vi "Remote_call_prep.vi"(3 "Vi Name in":string, 4 "Job Directory In":path, 5 "VI Directory":path) -> (0 "Vi Name out":string, 1 "Job Directory out":path, 2 "cancelled":bool)   [LabVIEW 2021]
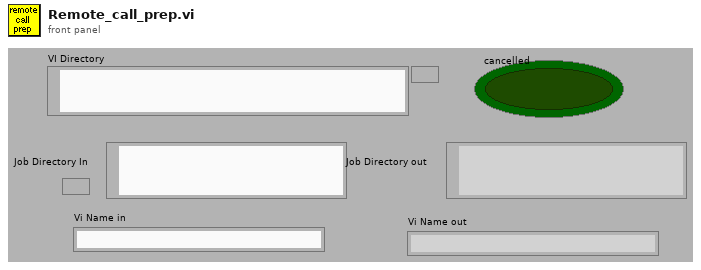
[diagram p1: front panel]
types:
  T1 = enum16{"Zero or one", "One", "Zero or more", "One or more"}
  T2 = enum32{"existing file", "new file", "new or existing file", "existing dir", "new dir", "new or existing dir", "existing file (use LLBs)", "new file (use LLBs)", "new or existing file (use LLBs)", "new or existing file or directory (use LLBs)"}
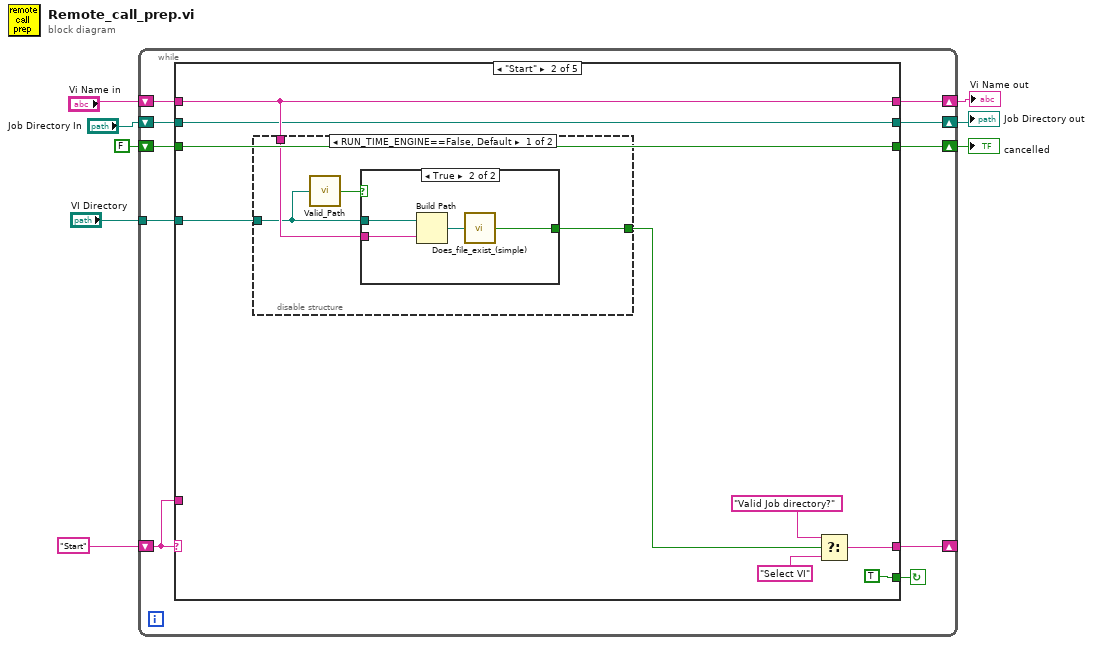
[diagram p0: block diagram]
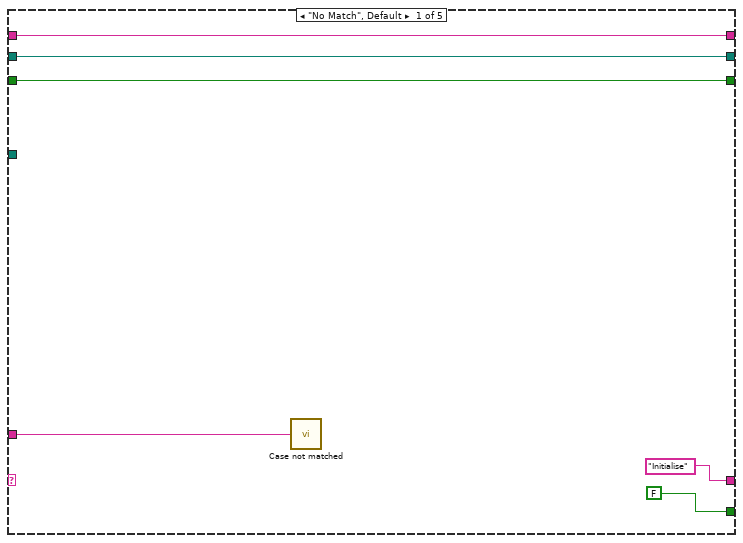
[diagram p2: hidden frame]
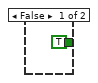
[diagram p3: hidden frame]
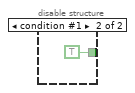
[diagram p4: hidden frame]
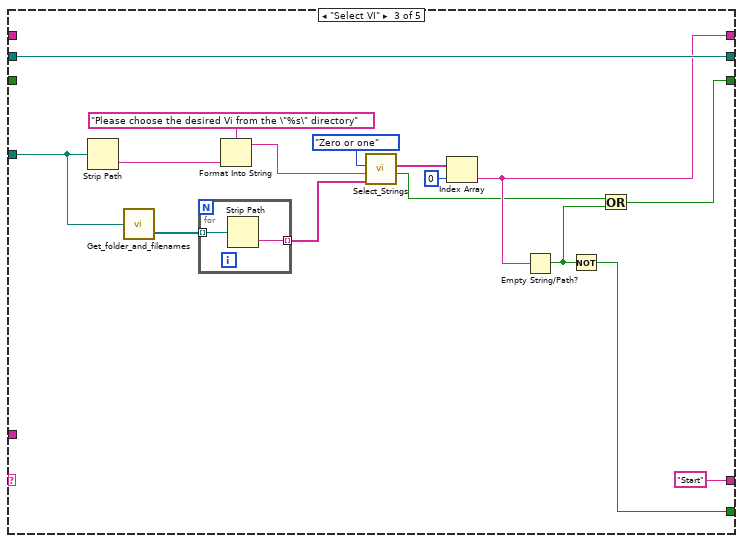
[diagram p5: hidden frame]
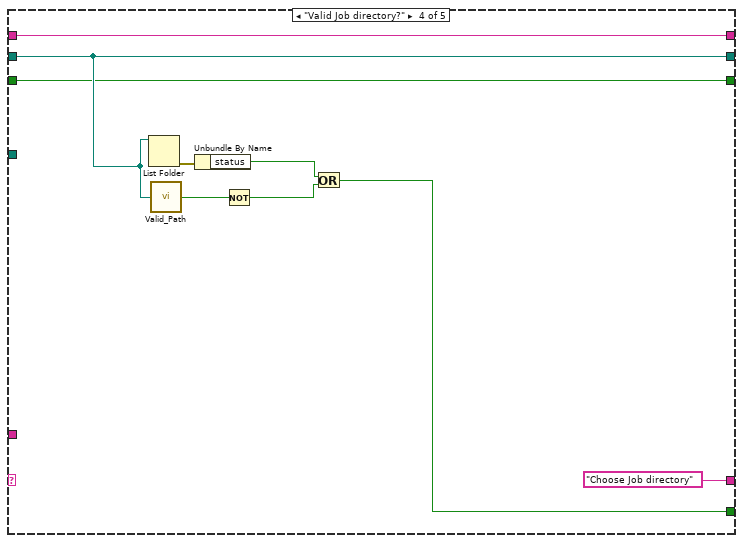
[diagram p6: hidden frame]
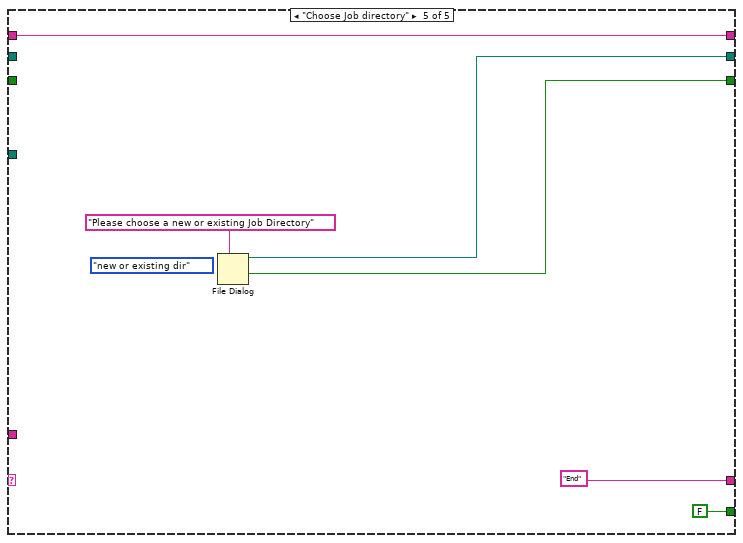
[diagram p7: hidden frame]
diagram:
  n1 = while {
    shift-left: "Start" -> [w16]
    shift-right: [w17] -> _
    tunnel: "VI Directory" -> [w15]
    shift-right: [w13] -> w5
    shift-left: "Vi Name in" -> [w14]
    shift-right: [w11] -> w2
    shift-left: "Job Directory In" -> [w12]
    shift-right: [w10] -> w3
    shift-left: FALSE ("cancelled") -> [w9]
    stop <- w18 continue-if-true
    n2 = case shown="\"Start\"" w16 {
      tunnel: [FALSE TRUE w47 w67 FALSE] -> w18
      tunnel: ["Initialise" w29 "Start" "Choose Job directory" "End"] -> w17
      tunnel: w16 -> [w20 _ _ _ _]
      tunnel: w15 -> [_ w26 w52 _ _]
      tunnel: w14 -> [w22 w28 _ w70 w76]
      tunnel: [w22 w28 w48 w70 w76] -> w13
      tunnel: w12 -> [w21 w27 w53 w68 _]
      tunnel: [w21 w27 w53 w68 w74] -> w11
      tunnel: [w19 w25 w44 w62 w73] -> w10
      tunnel: w9 -> [w19 w25 _ w62 _]
      frame "No Match", Default {
        n3 = call "Case not matched.vi"("Case Name not Matched"=w20) -> ()
      }
      frame "Start" {
        n4 = disable-structure shown="RUN_TIME_ENGINE==False, Default" {
          disable-tunnel: [w37 TRUE ("exists?")] -> w32
          disable-tunnel: w28 -> [w36 _]
          disable-tunnel: w26 -> [w35 _]
          frame condition #0 (active) {
            n5 = call "Valid_Path.vi"("Filename"=w35) -> ("Valid Path?"=w34:bool)
            n6 = case shown="True" w34 {
              tunnel: [TRUE ("exists?") w41] -> w37
              tunnel: w36 -> [_ w40]
              tunnel: w35 -> [_ w39]
              frame False {
              }
              frame True {
                n7 = Build Path(base path=w39, name or relative path=w40) -> (appended path=w42:path)
                n8 = call "Does_file_exist_(simple).vi"("Pathname"=w42) -> ("exists?"=w41:bool)
              }
            }
          }
          frame condition #1 {
          }
        }
        n9 = Select(t="Valid Job directory?", s=w32, f="Select VI") -> (s? t:f=w29:string)
      }
      frame "Select VI" {
        n10 = Strip Path(path=w52) -> (name=w51:string)  [unwired: 1 out]
        n11 = call "Get_folder_and_filenames.vi"("file path (dialog if empty)"=w52) -> ("Files"=w57:path[])  [unwired: 1 out]
        n12 = for {
          tunnel: w57 -> [w61] mode=indexing
          tunnel: [w60] -> w58 mode=indexing
          n13 = Strip Path(path=w61) -> (name=w60:string)  [unwired: 1 out]
        }
        n14 = Format Into String(format string="Please choose the desired Vi from the \"%s\" directory" ("Message"), w51) -> (resulting string=w49:string)  [unwired: 2 in, 1 out]
        n15 = call "Select_Strings.vi"("Available Ch names"=w58, "Message"=w49, "Selector mode"=T1."Zero or one") -> ("Cancel"=w45:bool, "Selected Channel Names"=w55:string[])  [unwired: 2 in, 2 out]
        n16 = Index Array(array=w55, index=0) -> (element=w48:string)
        n17 = Empty String/Path?(string/path=w48) -> (empty?=w46:bool)
        n18 = Not(x=w46) -> (.not. x?=w47:bool)
        n19 = Or(x=w45, y=w46) -> (x .or. y?=w44:bool)
      }
      frame "Valid Job directory?" {
        n20 = List Folder(path=w68) -> (error out=w66:errorcluster)  [unwired: 1 in, 5 out]
        n21 = call "Valid_Path.vi"("Filename"=w68) -> ("Valid Path?"=w65:bool)
        n22 = Unbundle By Name(w66) -> ("status"=w63:bool)
        n23 = Not(x=w65) -> (.not. x?=w64:bool)
        n24 = Or(x=w63, y=w64) -> (x .or. y?=w67:bool)
      }
      frame "Choose Job directory" {
        (unwired) T2."new or existing dir" ("select mode (2)")
        n25 = File Dialog(7:"Please choose a new or existing Job Directory" ("prompt")) -> (1:w73:bool, 3:w74:path)  [unwired: 1 in, 7 out]
      }
    }
  }
  "Vi Name out" <- w5
  "cancelled" <- w3
  "Job Directory out" <- w2
